vi "20-1.vi"() -> ()   [LabVIEW 2019, in "20.lvlib"]
uses:
  20.lvlib
panel:
  in  "Sample?":bool
  out "Lit":i16
  in  "Steps":i32
  out "Transformed Image":i16[][](graph)
  out "Initial Image":i16[][](graph)
  out "substring before match":string
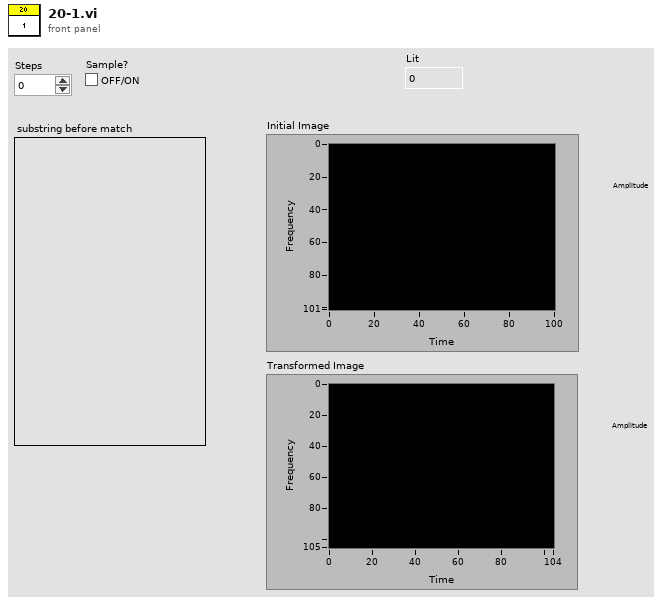
[diagram p1: front panel]
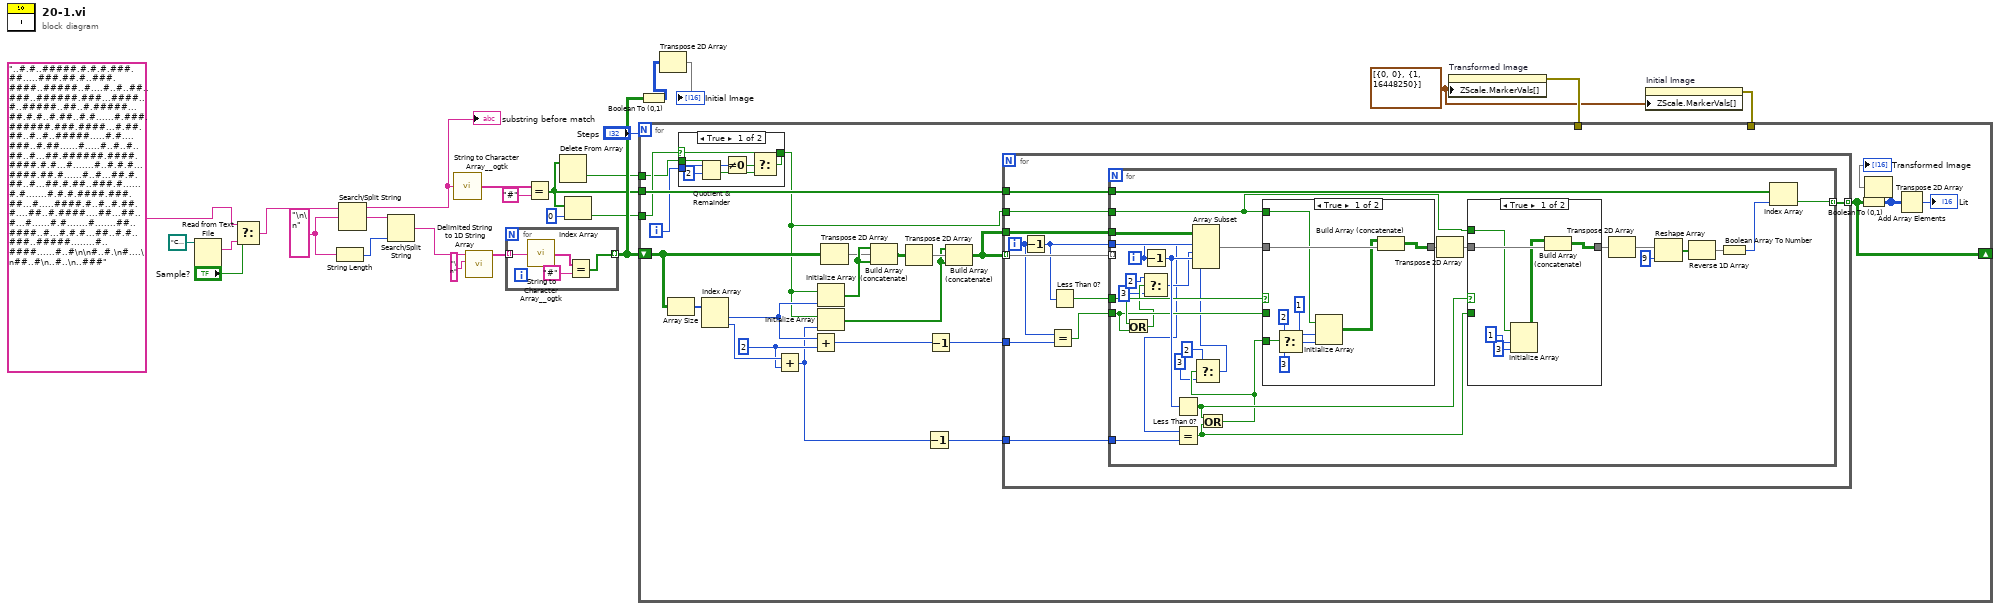
[diagram p0: block diagram]
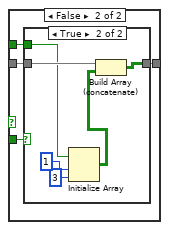
[diagram p2: hidden frame]
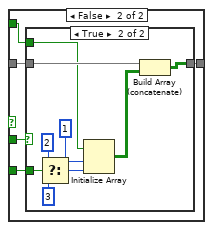
[diagram p4: hidden frame]
diagram:
  w13 = cluster{i16, u32}[] [{0, 0}, {1, 16448250}] ("Z Scale.Marker Values[]")
  w25 = "\n\n" ("search string/char (-)")
  n1 = Read from Text File(file (use dialog)=path "C:/Users/craig.walker/Documents/GitHub/lv2019-Advent-of-Code-2021/20/input.txt") -> (text=w9:string)  [unwired: 3 in, 3 out]
  n2 = Select(t="..#.#..#####.#.#.#.###.##.....###.##.#..###.####..#####..#....#..#..##..###..######.###...####..#..#####..##..#.#####...##.#.#..#.##..#.#......#.###.######.###.####...#.##.##..#..#..#####.....#.#....###..#.##......#.....#..#..#..##..#...##.######.####.####.#.#...#.......#..#.#.#...####.##.#......#..#...##.#.##..#...##.#.##..###.#......#.#.......#.#.#.####.###.##...#.....####.#..#..#.##.#....##..#.####....##...##..#...#......#.#.......#.......##..####..#...#.#.#...##..#.#..###..#####........#..####......#..#\n\n#..#.\n#....\n##..#\n..#..\n..###", s="Sample?", f=w9) -> (s? t:f=w7:string)
  n3 = String Length(string=w25) -> (length=w23:i32)
  n4 = Search/Split String(string=w7, search string/char (-)=w25) -> (substring before match=w19:string, match + rest of string=w24:string)  [unwired: 1 in, 1 out]
  "substring before match" <- w19
  n5 = Search/Split String(string=w24, offset (0)=w23) -> (match + rest of string=w22:string)  [unwired: 1 in, 2 out]
  n6 = call <userlib>:"String to Character Array__ogtk.vi"("Input String"=w19) -> ("Character Array"=w17:string[])
  n7 = call <vilib>:"Delimited String to 1D String Array.vi"("delimiter"="\n", "delimited string"=w22) -> ("string array"=w20:string[])  [unwired: 9 in]
  n8 = for {
    tunnel: w20 -> [w29] mode=indexing
    tunnel: [w26] -> w14 mode=indexing
    n9 = call <userlib>:"String to Character Array__ogtk.vi"("Input String"=w29) -> ("Character Array"=w27:string[])
    n10 = Equal?(x=w27, y="#") -> (x = y?=w26:bool[])
  }
  n11 = Equal?(x=w17, y="#") -> (x = y?=w2:bool[])
  n12 = Delete From Array(array=w2) -> (deleted portion=w1:bool)  [unwired: 2 in, 1 out]
  n13 = Index Array(array=w2, index=0) -> (element=w3:bool)
  n14 = Boolean To (0,1)(Boolean=w14) -> (0, 1=w11:i16[][])
  n15 = Transpose 2D Array(2D array=w11) -> (transposed array=→"Initial Image":i16[][])
  n16 = property on="Transformed Image" class="IntGraph (strict)"("ZScale.MarkerVals[]"=w13) -> (error out=w15:errorcluster)  [unwired: 2 in, 1 out]
  n17 = property on="Initial Image" class="IntGraph (strict)"("ZScale.MarkerVals[]"=w13) -> (error out=w12:errorcluster)  [unwired: 2 in, 1 out]
  n18 = for {
    N: "Steps" -> [_]
    tunnel: w2 -> [w47]
    shift-right: [w37] -> _
    shift-left: w14 -> [w40]
    tunnel: w15 -> [_]
    tunnel: w12 -> [_]
    tunnel: w3 -> [w33]
    tunnel: w1 -> [w31]
    i -> [w32]
    w43 = 2 ("y")
    n19 = Array Size(array=w40) -> (size(s)=w53:i32[])
    n20 = case shown="True" w33 {
      selector: w33 -> [w137 w142]
      tunnel: w32 -> [w141 _]
      tunnel: [w135 w142] -> w30
      tunnel: w31 -> [w136 _]
      frame True {
        n21 = Quotient & Remainder(x=w141, y=2) -> (x-y*floor(x/y)=w139:i32)  [unwired: 1 out]
        n22 = Not Equal To 0?(x=w139) -> (x != 0?=w138:bool)
        n23 = Select(t=w137, s=w138, f=w136) -> (s? t:f=w135:bool)
      }
      frame False {
      }
    }
    n24 = Index Array(array=w53) -> (element #1=w44:i32, element #2=w46:i32)  [unwired: 2 in]
    n25 = Add(x=w46, y=w43) -> (x+y=w41:i32)
    n26 = Add(x=w44, y=w43) -> (x+y=w42:i32)
    n27 = Initialize Array(w30, w44) -> (w52:bool[])
    n28 = Initialize Array(w30, w41) -> (w45:bool[])
    n29 = Transpose 2D Array(2D array=w40) -> (transposed array=w48:bool[][])
    n30 = Build Array (concatenate)(w52, w48, w52) -> (w51:bool[][])
    n31 = Transpose 2D Array(2D array=w51) -> (transposed array=w50:bool[][])
    n32 = Decrement(x=w41) -> (x-1=w38:i32)
    n33 = Decrement(x=w42) -> (x-1=w39:i32)
    n34 = Build Array (concatenate)(w45, w50, w45) -> (w49:bool[][])
    n35 = for {
      tunnel: w49 -> [w64] mode=indexing
      tunnel: w49 -> [w63]
      tunnel: w47 -> [w62]
      tunnel: w39 -> [w60]
      tunnel: w38 -> [w59]
      tunnel: [w56] -> w37 mode=indexing
      tunnel: w30 -> [w54]
      i -> [w55]
      n36 = Decrement(x=w55) -> (x-1=w61:i32)
      n37 = Equal?(x=w55, y=w60) -> (x = y?=w57:bool)
      n38 = Less Than 0?(x=w61) -> (x < 0?=w58:bool)
      n39 = for {
        tunnel: w64 -> [_] mode=indexing
        tunnel: w63 -> [w93]
        tunnel: w62 -> [w89]
        tunnel: w61 -> [w92]
        tunnel: w59 -> [w86]
        tunnel: w58 -> [w80]
        tunnel: w57 -> [w79]
        tunnel: [w82] -> w56 mode=indexing
        tunnel: w54 -> [w65]
        i -> [w66]
        n40 = Or(x=w80, y=w79) -> (x .or. y?=w78:bool)
        n41 = Decrement(x=w66) -> (x-1=w87:i32)
        n42 = Select(t=2 ("length"), s=w78, f=3) -> (s? t:f=w77:i32)
        n43 = Less Than 0?(x=w87) -> (x < 0?=w84:bool)
        n44 = Equal?(x=w66, y=w86) -> (x = y?=w83:bool)
        n45 = Or(x=w84, y=w83) -> (x .or. y?=w75:bool)
        n46 = Select(t=2 ("length"), s=w75, f=3) -> (s? t:f=w72:i32)
        n47 = Array Subset(array=w93, index (row)=w92, length (row)=w77, index (col)=w87, length (col)=w72) -> (w71:bool[][])
        n48 = case shown="True" w80 {
          tunnel: w71 -> [w119 w124]
          tunnel: [w118 w123] -> w70
          tunnel: w75 -> [w113 w122]
          tunnel: w79 -> [_ w121]
          tunnel: w65 -> [w111 w120]
          frame True {
            n49 = Select(t=2, s=w113, f=3) -> (s? t:f=w114:i32)
            n50 = Initialize Array(w111, 1, w114) -> (w112:bool[][])
            n51 = Build Array (concatenate)(w112, w119) -> (w118:bool[][])
          }
          frame False {
            n52 = case shown="True" w121 {
              tunnel: w124 -> [w125 w134]
              tunnel: [w125 w133] -> w123
              tunnel: w122 -> [_ w129]
              tunnel: w120 -> [_ w132]
              frame False {
              }
              frame True {
                n53 = Select(t=2, s=w129, f=3) -> (s? t:f=w126:i32)
                n54 = Initialize Array(w132, 1, w126) -> (w131:bool[][])
                n55 = Build Array (concatenate)(w134, w131) -> (w133:bool[][])
              }
            }
          }
        }
        n56 = Transpose 2D Array(2D array=w70) -> (transposed array=w69:bool[][])
        n57 = case shown="True" w84 {
          tunnel: w69 -> [w99 w103]
          tunnel: [w98 w102] -> w85
          tunnel: w83 -> [_ w101]
          tunnel: w65 -> [w95 w100]
          frame True {
            n58 = Initialize Array(w95, 1, 3 ("dimension size")) -> (w94:bool[][])
            n59 = Build Array (concatenate)(w94, w99) -> (w98:bool[][])
          }
          frame False {
            n60 = case shown="True" w101 {
              tunnel: w103 -> [w104 w110]
              tunnel: [w104 w109] -> w102
              tunnel: w100 -> [_ w105]
              frame False {
              }
              frame True {
                n61 = Initialize Array(w105, 1, 3 ("dimension size")) -> (w106:bool[][])
                n62 = Build Array (concatenate)(w110, w106) -> (w109:bool[][])
              }
            }
          }
        }
        n63 = Transpose 2D Array(2D array=w85) -> (transposed array=w68:bool[][])
        n64 = Reshape Array(w68, 9 ("dimension size")) -> (w90:bool[])
        n65 = Reverse 1D Array(array=w90) -> (reversed array=w67:bool[])
        n66 = Boolean Array To Number(Boolean array=w67) -> (number=w88:u16)
        n67 = Index Array(array=w89, index=w88) -> (element=w82:bool)
      }
    }
    n68 = Boolean To (0,1)(Boolean=w37) -> (0, 1=w35:i16[][])
    n69 = Transpose 2D Array(2D array=w35) -> (transposed array=→"Transformed Image":i16[][])
    n70 = Add Array Elements(numeric array=w35) -> (sum=→"Lit":i16)
  }
